vi "OutputIV.vi"(5 "Sampling Rate:":dbl=5000.0, 6 "MessageQueues":T1, 7 "MonitorTask":refnum<k21>, 8 "BiasChannel":refnum<k21>, 9 "Bias Voltage (mV)":string, 10 "TraceTime":dbl, 11 "frequency":dbl) -> ()   [LabVIEW 2024]
uses:
  MessageQueues.ctl
  <vilib>/httpClient/ClientHandle.ctl
  <vilib>/Platform/TimedLoop/XDataNode/timing_clust.ctl
  <vilib>/Platform/TimedLoop/XDataNode/nitl_modes.ctl
  <vilib>/Platform/TimedLoop/XDataNode/wakeup.ctl
  <vilib>/DAQmx/write.llb/DAQmx Write (Analog 1D Wfm NChan NSamp).vi
  <vilib>/DAQmx/configure/timing.llb/DAQmx Timing (Sample Clock).vi
  <vilib>/DAQmx/miscellaneous.llb/DAQmx Fill In Error Info.vi
  <vilib>/Platform/TimedLoop/XDataNode/XDataNode.xnode
  <resource>/objmgr/daqmx.rc
  <vilib>/measure/NI_MABase.lvlib
  <vilib>/Platform/TimedLoop/XDataNode/XDNodeRunTimeDep.lvlib
  <vilib>/httpClient/LabVIEWHTTPClient.lvlib
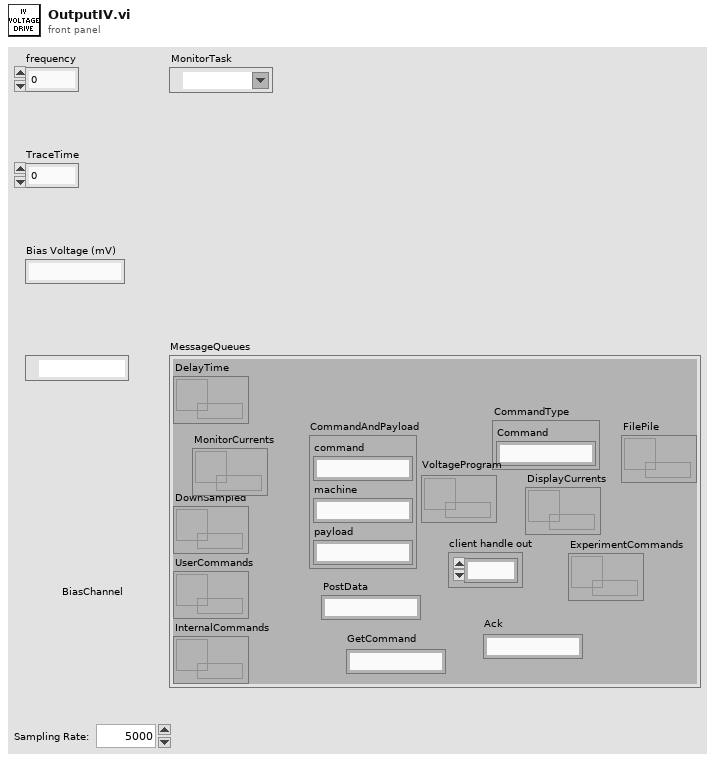
[diagram p1: front panel]
types:
  T1 = typedef "MessageQueues.ctl" = cluster{"DelayTime":refnum<queue>, "DownSampled":refnum<queue>, "UserCommands":refnum<queue>, "InternalCommands":refnum<queue>, "CommandType":cluster{"Command":string}, "CommandAndPayload":cluster{"command":string, "machine":string, "payload":string}, "client handle out":T2, "PostData":string, "GetCommand":string, "Ack":string, "VoltageProgram":refnum<queue>, "ExperimentCommands":refnum<queue>, "DisplayCurrents":refnum<queue>, "MonitorCurrents":refnum<queue>, "FilePile":refnum<queue>}
  T2 = typedef "LabVIEWHTTPClient.lvlib/ClientHandle.ctl" = refnum<k1>
  T3 = typedef "XDNodeRunTimeDep.lvlib/timing_clust.ctl" = cluster{"Expected End [f-1]":u64, "Actual End [f-1]":u64, "Finished Late? [f-1]":bool, "Expected End [i-1]":u64, "Actual End [i-1]":u64, "Finished Late? [i-1]":bool, "Expected Start [i]":u64, "Actual Start [i]":u64, "Expected Start [f]":u64, "Actual Start [f]":u64, "Source Name":string, "Structure Name":string, "Period":i64, "Deadline":i64, "Offset":i64, "Start":i64, "Priority":i32, "Timeout":i32, "Mode":T4, "Wakeup Reason":T5, "Error":errorcluster, "Source Type":string, "Secondary Source Type":string, "Global End Time":u64, "Global Start Time":u64, "Frame Duration":u64, "Iteration Duration":u64, "Assigned CPU":i32, "I/O Scan Engine Mode":u32}
  T4 = typedef "XDNodeRunTimeDep.lvlib/nitl_modes.ctl" = enum32{"No Change", "Process missed periods, maintain original phase", "Discard missed periods, maintain original phase", "Process missed periods, ignore original phase", "Discard missed periods, ignore original phase"}
  T5 = typedef "XDNodeRunTimeDep.lvlib/wakeup.ctl" = enum32{"Normal", "Aborted", "Asynchronous wakeup", "Timing source error", "Timed loop error", "Timeout"}
  T6 = enum16{"Sine Wave", "Triangle Wave", "Square Wave", "Sawtooth Wave"}
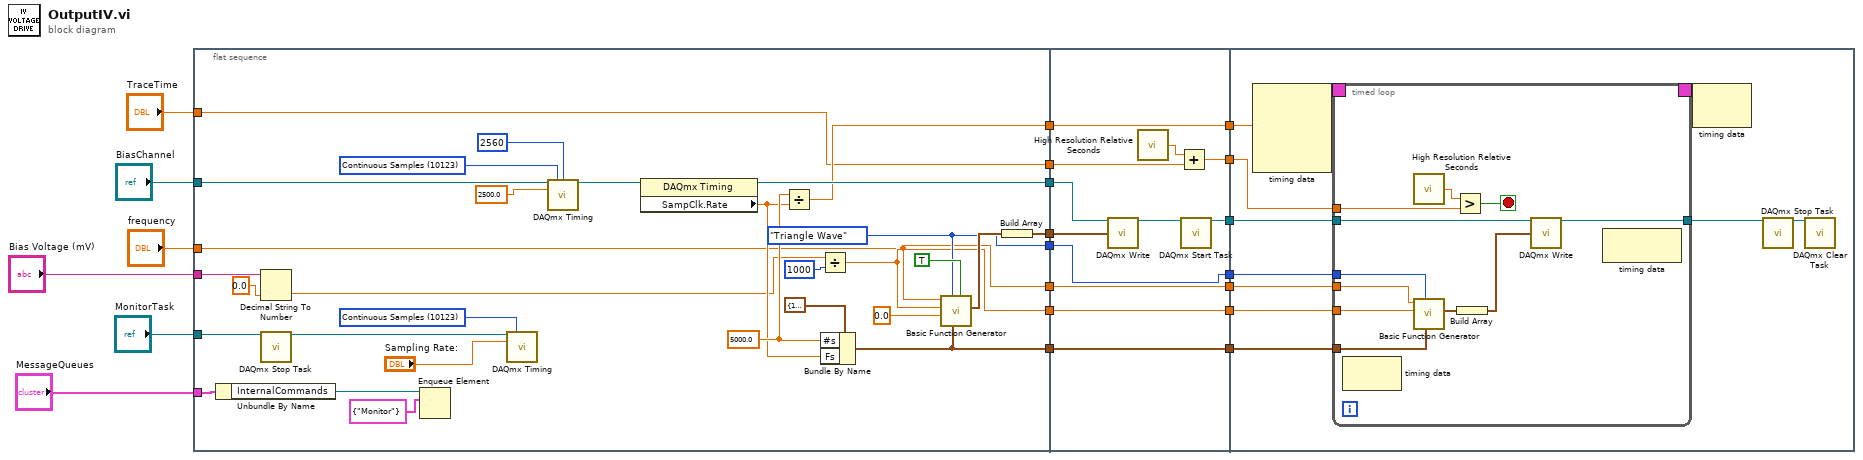
[diagram p0: block diagram]
diagram:
  n1 = flat-sequence {
    tunnel: [w43] -> w21
    tunnel: [w48] -> w20
    tunnel: [w31] -> w19
    tunnel: [w42] -> w18
    tunnel: [w32] -> w17
    tunnel: [w35] -> w16
    tunnel: [w41] -> w15
    tunnel: [w37] -> w14
    tunnel: "Bias Voltage (mV)" -> [w33]
    tunnel: "frequency" -> [w32]
    tunnel: "TraceTime" -> [w31]
    tunnel: "MessageQueues" -> [w28]
    tunnel: "BiasChannel" -> [w29]
    tunnel: "MonitorTask" -> [w26]
    tunnel: [w59] -> w9
    tunnel: w21 -> [w61]
    tunnel: w20 -> [w62]
    tunnel: w19 -> [w63]
    tunnel: [w58] -> w8
    tunnel: w18 -> [w58]
    tunnel: w17 -> [w57]
    tunnel: [w57] -> w7
    tunnel: [w56] -> w6
    tunnel: w16 -> [w56]
    tunnel: w15 -> [w55]
    tunnel: [w55] -> w4
    tunnel: [w54] -> w3
    tunnel: w14 -> [w54]
    tunnel: [w52] -> w5
    tunnel: w9 -> [w71]
    tunnel: w8 -> [w74]
    tunnel: w7 -> [w73]
    tunnel: w6 -> [w72]
    tunnel: w5 -> [w70]
    tunnel: w4 -> [w68]
    tunnel: w3 -> [w65]
    frame #0 {
      w27 = 10123 items=["Finite Samples"=10178, "Continuous Samples"=10123, "Hardware Timed Single Point"=12522] ("sample mode")
      w39 = 5000.0 ("#s")
      w42 = T6."Triangle Wave" ("signal type")
      w51 = 10123 items=["Finite Samples"=10178, "Continuous Samples"=10123, "Hardware Timed Single Point"=12522] ("sample mode")
      n2 = Unbundle By Name(w28) -> ("InternalCommands"=w23:refnum<queue>)
      n3 = Decimal String To Number(string=w33, default (0L)=0.0) -> (number=w36:dbl)  [unwired: 1 in, 1 out]
      n4 = call <vilib>:"DAQmx Stop Task.vi"("task/channels in"=w26) -> ("task out"=w25:refnum<k21>)  [unwired: 13 in, 1 out]
      n5 = Enqueue Element(queue=w23, element=cluster{"Command":string} {"Command"="Monitor"}) -> ()  [unwired: 2 in, 3 out]
      n6 = call-poly <vilib>:"DAQmx Timing.vi"("task/channels in"=w25, "sample mode"=w27, "rate"="Sampling Rate:") -> ()  [unwired: 11 in, 2 out]
      n7 = call-poly <vilib>:"DAQmx Timing.vi"("task/channels in"=w29, "sample mode"=w51, "samples per channel"=2560, "rate"=2500.0) -> ("task out"=w49:refnum<k21>)  [unwired: 10 in, 1 out]
      n8 = property class="DAQmx Timing"(reference=w49) -> (reference out=w48:refnum<k21>, "SampClk.Rate"=w38:dbl)  [unwired: 1 in, 1 out]
      n9 = Divide(x=w39, y=w38) -> (x/y=w37:dbl)
      n10 = Divide(x=w36, y=1000) -> (x/y=w35:dbl)
      n11 = Bundle By Name(cluster=cluster{"Fs":dbl, "#s":dbl} {"Fs"=1000.0, "#s"=1000.0} ("sampling info"), "#s"=w39, "Fs"=w38) -> (w41:cluster{"Fs":dbl, "#s":dbl})
      n12 = call <vilib>:"Basic Function Generator.vi"("reset signal"=TRUE, "sampling info"=w41, "signal type"=w42, "phase"=0.0, "amplitude"=w35, "frequency"=w32) -> ("signal out"=w47:waveform(dbl))  [unwired: 3 in, 2 out]
      n13 = Build Array(w47) -> (w43:waveform(dbl)[])
    }
    frame #1 {
      n14 = call-poly <vilib>:"DAQmx Write.vi"("task/channels in"=w62, "data"=w61) -> ("task out"=w60:refnum<k21>)  [unwired: 11 in, 2 out]
      n15 = call <vilib>:"High Resolution Relative Seconds.vi"() -> ("relative seconds"=w53:dbl)
      n16 = Add(x=w53, y=w63) -> (x+y=w52:dbl)
      n17 = call <vilib>:"DAQmx Start Task.vi"("task/channels in"=w60) -> ("task out"=w59:refnum<k21>)  [unwired: 13 in, 1 out]
    }
    frame #2 {
      n18 = node-c288(w65) -> (w67:T3)  [unwired: 3 in]
      n19 = timed-loop {
        tunnel: w74 -> [w85]
        tunnel: w73 -> [w84]
        tunnel: w72 -> [w83]
        tunnel: w71 -> [w80]
        tunnel: w70 -> [w78]
        tunnel: [w76] -> w69
        tunnel: w68 -> [w75]
        timing: w67 -> [_]
        timing-out: [_] -> w66
        stop <- w77 stop-if-true
        n20 = node-c288() -> ()  [unwired: 1 in, 1 out]
        n21 = call <vilib>:"High Resolution Relative Seconds.vi"() -> ("relative seconds"=w79:dbl)
        n22 = call <vilib>:"Basic Function Generator.vi"("sampling info"=w75, "signal type"=w85, "amplitude"=w83, "frequency"=w84) -> ("signal out"=w82:waveform(dbl))  [unwired: 5 in, 2 out]
        n23 = Greater?(x=w79, y=w78) -> (0:w77:bool)
        n24 = Build Array(w82) -> (w81:waveform(dbl)[])
        n25 = call-poly <vilib>:"DAQmx Write.vi"("task/channels in"=w80, "data"=w81) -> ("task out"=w76:refnum<k21>)  [unwired: 11 in, 2 out]
        n26 = node-c288() -> ()  [unwired: 1 in, 1 out]
      }
      n27 = node-c288(w66) -> ()  [unwired: 1 out]
      n28 = call <vilib>:"DAQmx Stop Task.vi"("task/channels in"=w69) -> ("task out"=w64:refnum<k21>)  [unwired: 13 in, 1 out]
      n29 = call <vilib>:"DAQmx Clear Task.vi"("task in"=w64) -> ()  [unwired: 14 in, 1 out]
    }
  }
